vi "LMS on SW Map 2h.vi"(8 "SW Map In":i32[][](array[numeric]), 11 "LMS Vector":dbl[](array[numeric])) -> (3 "SW Map Out":i32[][](array[numeric]))   [LabVIEW 2014]
panel:
  out "LMS Vector Check":dbl[](array[numeric])
  out "Test SW Map Out of y":dbl[](array[numeric])
  out "Test SW Map Out of x":dbl[](array[numeric])
  # "Inputs:"
  # "Outputs:"
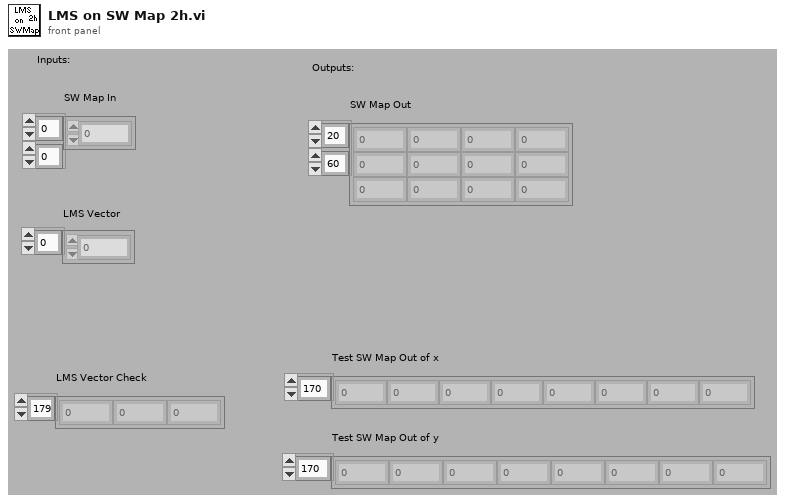
[diagram p1: front panel]
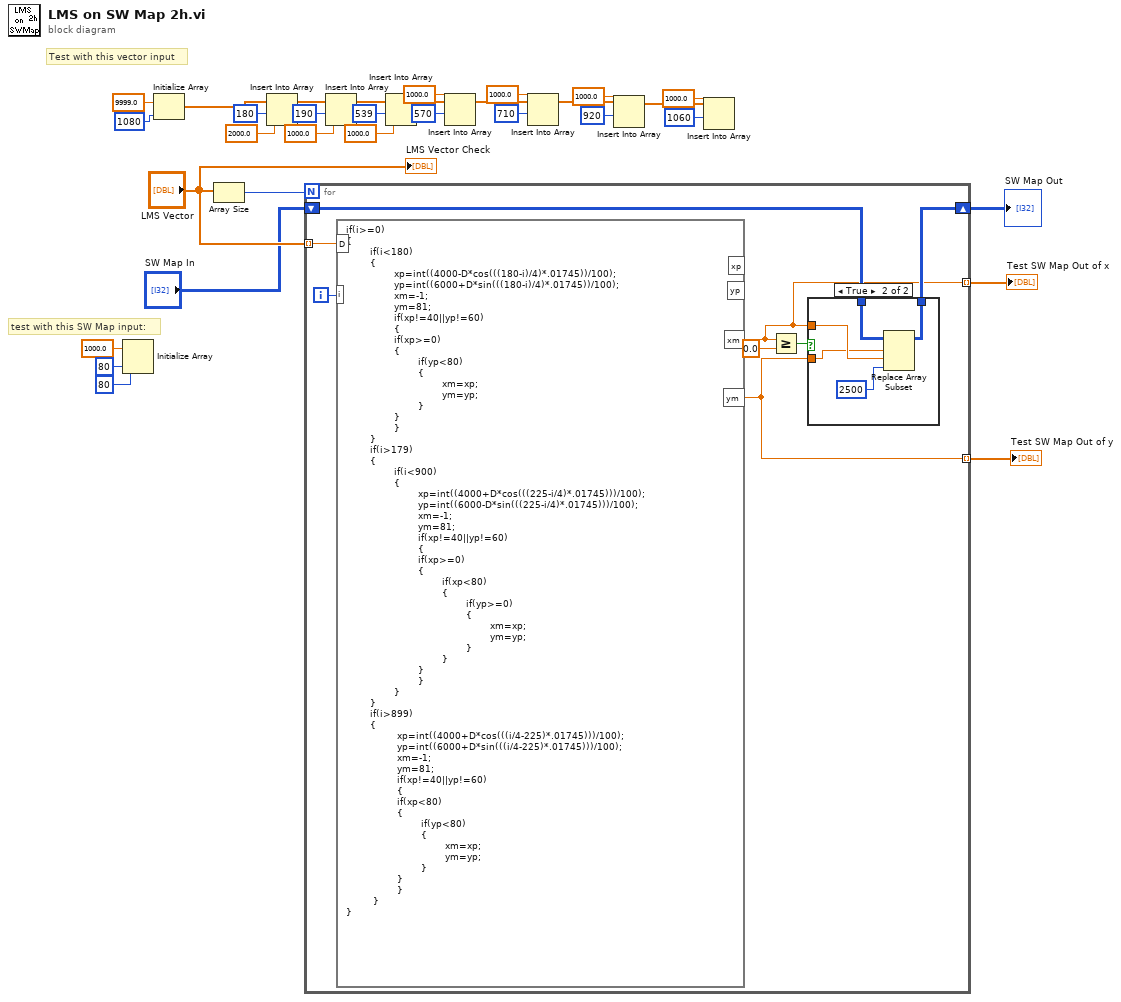
[diagram p0: block diagram]
diagram:
  # "test with this SW Map input:"
  # "Test with this vector input"
  n1 = Initialize Array(1000.0 ("element"), 80 ("dimension size"), 80 ("dimension size")) -> ()  [unwired: 1 out]
  n2 = Initialize Array(9999.0 ("element"), 1080 ("dimension size")) -> (w31:dbl[])
  n3 = Array Size(array="LMS Vector") -> (size(s)=w29:i32)
  n4 = Insert Into Array(array=w31, index=180 ("index (row)"), new element=2000.0 ("new element/subarray")) -> (w3:dbl[])
  n5 = for {
    N: w29 -> [_]
    tunnel: "LMS Vector" -> [w40] mode=indexing
    shift-right: [w35] -> w9
    shift-left: "SW Map In" -> [w38]
    tunnel: [w34] -> w8 mode=indexing
    tunnel: [w33] -> w7 mode=indexing
    i -> [w39]
    n6 = formula code="if(i>=0) \n{\n        if(i<180)\n        {\n                xp=int((4000-D*cos(((180-i)/4)*.01745))/100);\n                yp=int((6000+D*sin(((180-i)/4)*.01745))/100);\n                xm=-1;\n                ym=81;\n                if(xp!=40||yp!=60)\n                {\n                if(xp>=0)\n                {\n                        if(yp<80)\n                        {\n                                xm=xp;\n                                ym=yp;\n                        }\n                }\n                }\n        }\n        if(i>179)\n        {\n                if(i<900)\n                {\n                        xp=int((4000+D*cos(((225-i/4)*.01745)))/100);\n                        yp=int((6000-D*sin(((225-i/4)*.01745)))/100);\n                        xm=-1;\n                        ym=81;\n                        if(xp!=40||yp!=60)\n                        {\n                        if(xp>=0)\n                        {\n                                if(xp<80)\n                                {\n                                        if(yp>=0)\n                                        {\n                                                xm=xp;\n                                                ym=yp;\n                                        }\n                                }\n                        }\n                        }\n                }\n        }\n        if(i>899)\n        {\n                 xp=int((4000+D*cos(((i/4-225)*.01745)))/100);\n                 yp=int((6000+D*sin(((i/4-225)*.01745)))/100);\n                 xm=-1;\n                 ym=81;\n                 if(xp!=40||yp!=60)\n                 {\n                 if(xp<80)\n                 {\n                         if(yp<80)\n                         {\n                                 xm=xp;\n                                 ym=yp;\n                         }\n                 }\n                 }\n         }\n}"("D"=w40, "i"=w39) -> ("xm"=w33:dbl, "ym"=w34:dbl)  [unwired: 2 out]
    n7 = Greater Or Equal?(x=w33, y=0.0) -> (x >= y?=w36:bool)
    n8 = case shown="True" w36 {
      tunnel: w38 -> [w41 w46]
      tunnel: [w41 w45] -> w35
      tunnel: w34 -> [_ w42]
      tunnel: w33 -> [_ w43]
      frame False {
      }
      frame True {
        n9 = Replace Array Subset(array=w46, new element=2500, index (row)=w42, index (col)=w43) -> (w45:i32[][])
      }
    }
  }
  "SW Map Out" <- w9
  "Test SW Map Out of x" <- w7
  "Test SW Map Out of y" <- w8
  n10 = Insert Into Array(array=w3, index=190, new element=1000.0 ("new element/subarray")) -> (w24:dbl[])
  n11 = Insert Into Array(array=w24, index=539, new element=1000.0 ("new element/subarray")) -> (w21:dbl[])
  n12 = Insert Into Array(array=w21, index=570, new element=1000.0 ("new element/subarray")) -> (w18:dbl[])
  n13 = Insert Into Array(array=w18, index=710, new element=1000.0 ("new element/subarray")) -> (w15:dbl[])
  n14 = Insert Into Array(array=w15, index=920, new element=1000.0 ("new element/subarray")) -> (w12:dbl[])
  n15 = Insert Into Array(array=w12, index=1060, new element=1000.0 ("new element/subarray")) -> ()  [unwired: 1 out]
  "LMS Vector Check" <- "LMS Vector"
